vi "Event Info to Links.vi"(11 "Event Info":T2[](array[typedef])) -> (1 "Request With Reply Links":T1[](array[typedef]), 2 "Broadcast Links":T1[](array[typedef]), 3 "Request Links":T1[](array[typedef]))   [LabVIEW 2021, in "TAF Proj Document Type.lvlib" / "Project Parser.lvlib"]
uses:
  <vilib>/Wovalab/AntiDoc/Document Type/Add-ons/LabVIEW TAF Project/Project Parser/Project Parser.lvlib
  <vilib>/Wovalab/AntiDoc/Document Type/Add-ons/LabVIEW TAF Project/Project Parser/Dqmh Event Info--cluster.ctl
  <vilib>/Wovalab/AntiDoc/Document Type/Add-ons/LabVIEW TAF Project/Project Parser/Dqmh Event Type--enum.ctl
  <vilib>/Wovalab/AntiDoc/Document Type/Add-ons/LabVIEW TAF Project/Project Parser/Dqmh Event Links--cluster.ctl
  <vilib>/picture/picture.llb/imagedata.ctl
  <vilib>/Wovalab/AntiDoc/Document Type/Add-ons/LabVIEW TAF Project/Project Parser/Dqmh Event Callers--cluster.ctl
  <vilib>/Wovalab/AntiDoc/Utilities/Utilities.lvlib
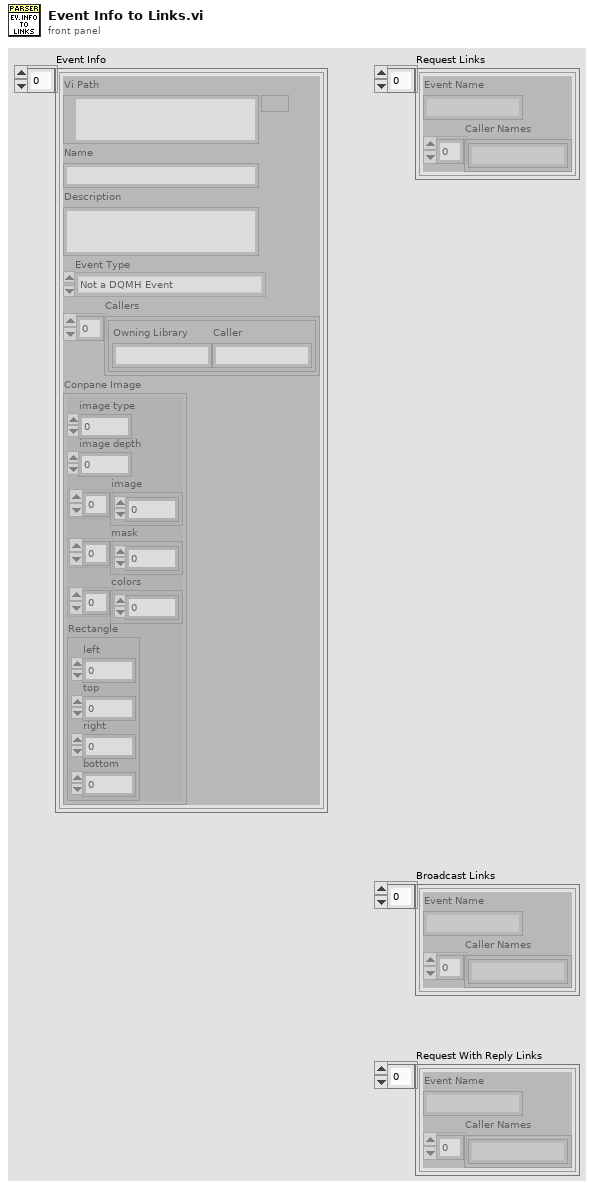
[diagram p1: front panel]
types:
  T1 = typedef "TAF Proj Document Type.lvlib/Project Parser.lvlib/Dqmh Event Callers--cluster.ctl" = cluster{"Event Name":string, "Caller Names":string[]}
  T2 = typedef "TAF Proj Document Type.lvlib/Project Parser.lvlib/Dqmh Event Info--cluster.ctl" = cluster{"Vi Path":path, "Name":string, "Description":string, "Event Type":T3, "Callers":T4[], "Conpane Image":T5}
  T3 = typedef "TAF Proj Document Type.lvlib/Project Parser.lvlib/Dqmh Event Type--enum.ctl" = enum16{"Not a DQMH Event", "Request", "Request And Wait For Reply", "Broadcast"}
  T4 = typedef "TAF Proj Document Type.lvlib/Project Parser.lvlib/Dqmh Event Links--cluster.ctl" = cluster{"Owning Library":string, "Caller":string}
  T5 = typedef "imagedata.ctl" = cluster{"image type":i32, "image depth":i32, "image":u8[], "mask":u8[], "colors":u32[], "Rectangle":cluster{"left":i16, "top":i16, "right":i16, "bottom":i16}}
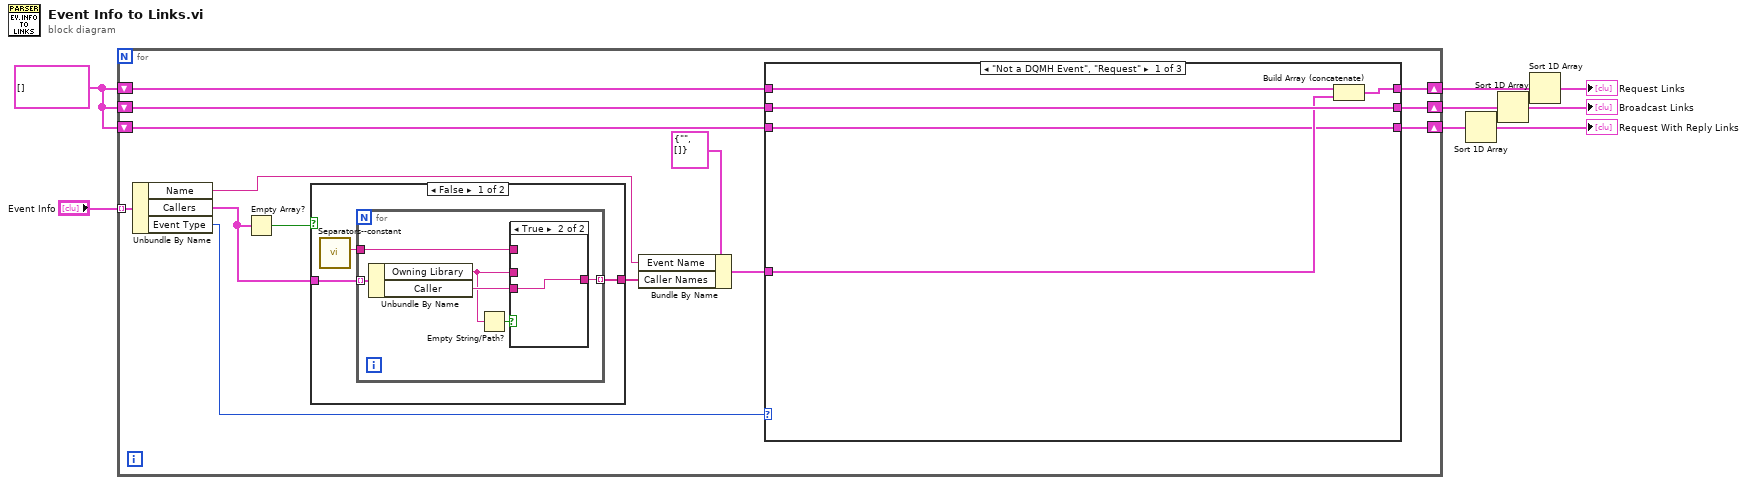
[diagram p0: block diagram]
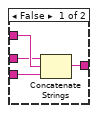
[diagram p2: hidden frame]
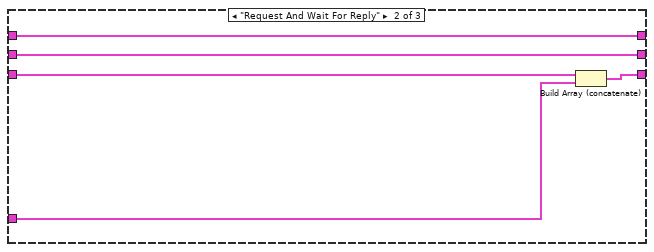
[diagram p4: hidden frame]
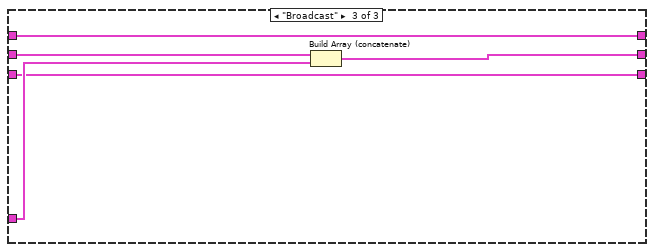
[diagram p5: hidden frame]
diagram:
  w5 = T1[] [] ("appended array")
  n1 = for {
    tunnel: "Event Info" -> [w22] mode=indexing
    shift-right: [w19] -> w7
    shift-left: w5 -> [w20]
    shift-right: [w18] -> w6
    shift-left: w5 -> [w17]
    shift-right: [w9] -> w4
    shift-left: w5 -> [w10]
    n2 = Unbundle By Name(w22) -> ("Name"=w14:string, "Callers"=w13:T4[], "Event Type"=w21:T3)
    n3 = Empty Array?(array=w13) -> (empty?=w15:bool)
    n4 = case shown="False" w15 {
      tunnel: w13 -> [w25 _]
      tunnel: [w24 _] -> w16
      frame False {
        n5 = call <vilib>:"Separators--constant.vi"() -> ("Caller Lib Owner Separator"=w23:string)  [unwired: 10 in, 1 out]
        n6 = for {
          tunnel: w25 -> [w31] mode=indexing
          tunnel: [w29] -> w24 mode=indexing
          tunnel: w23 -> [w28]
          n7 = Unbundle By Name(w31) -> ("Owning Library"=w27:string, "Caller"=w30:string)
          n8 = Empty String/Path?(string/path=w27) -> (empty?=w26:bool)
          n9 = case shown="True" w26 {
            tunnel: w30 -> [w35 w36]
            tunnel: [w34 w36] -> w29
            tunnel: w28 -> [w33 _]
            tunnel: w27 -> [w32 _]
            frame False {
              n10 = Concatenate Strings(w32, w33, w35) -> (w34:string)
            }
            frame True {
            }
          }
        }
      }
      frame True {
      }
    }
    n11 = Bundle By Name(cluster=T1 {"Event Name"="", "Caller Names"=[]} ("Event Callers"), "Event Name"=w14, "Caller Names"=w16) -> (w12:T1)
    n12 = case shown="\"Not a DQMH Event\", \"Request\"" w21 {
      tunnel: w20 -> [w41 w46 w51]
      tunnel: [w40 w46 w51] -> w19
      tunnel: [w39 w45 w49] -> w18
      tunnel: w17 -> [w39 w45 w50]
      tunnel: w12 -> [w38 w43 w48]
      tunnel: w10 -> [w37 w44 w47]
      tunnel: [w37 w42 w47] -> w9
      frame "Not a DQMH Event", "Request" {
        n13 = Build Array (concatenate)(w41, w38) -> (w40:T1[])
      }
      frame "Request And Wait For Reply" {
        n14 = Build Array (concatenate)(w44, w43) -> (w42:T1[])
      }
      frame "Broadcast" {
        n15 = Build Array (concatenate)(w50, w48) -> (w49:T1[])
      }
    }
  }
  n16 = Sort 1D Array(array=w4) -> (sorted array=→"Request With Reply Links":T1[])
  n17 = Sort 1D Array(array=w6) -> (sorted array=→"Broadcast Links":T1[])
  n18 = Sort 1D Array(array=w7) -> (sorted array=→"Request Links":T1[])
